vi "Multiplicate Number.vi"(8 "error in (no error)":errorcluster, 9 "Number 2":dbl, 10 "Number 1":dbl, 11 "Multiplication Actor in":refnum<class "Multiplication Actor.lvclass">) -> (0 "error out":errorcluster, 3 "Multiplication Actor out":refnum<class "Multiplication Actor.lvclass">)   [LabVIEW 2015, in "Multiplication Actor.lvclass"]
uses:
  Multiplication Actor.lvclass
  <vilib>/ActorFramework/Actor/Actor.lvclass/Actor.ctl
  Calculator Actor/Calculator Actor Messages/Update Multiplication Result Ref Msg/Update Multiplication Result Ref Msg.lvclass/Update Multiplication Result Ref Msg.ctl
  <vilib>/ActorFramework/Message Enqueuer/Message Enqueuer.lvclass/Message Enqueuer.ctl
  <vilib>/ActorFramework/Message Enqueuer/Enqueue.vi
  <vilib>/ActorFramework/Message Priority Queue/Priority Enqueue.vi
  Calculator Actor/Calculator Actor Messages/Update Multiplication Result Ref Msg/Update Multiplication Result Ref Msg.lvclass
  <vilib>/ActorFramework/Actor/Actor.lvclass
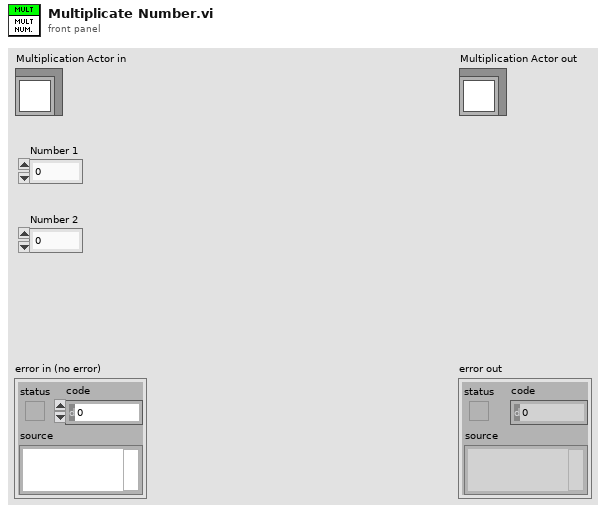
[diagram p1: front panel]
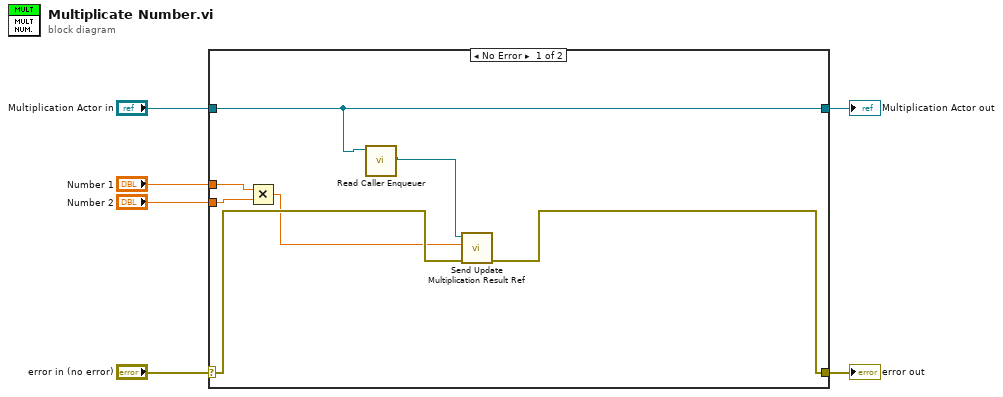
[diagram p0: block diagram]
diagram:
  n1 = case shown="No Error" "error in (no error)" {
    selector: "error in (no error)" -> [w13 w15]
    tunnel: [w12 w15] -> w5
    tunnel: [w8 w14] -> w3
    tunnel: "Multiplication Actor in" -> [w8 w14]
    tunnel: "Number 1" -> [w11 _]
    tunnel: "Number 2" -> [w10 _]
    frame No Error {
      n2 = Multiply(x=w11, y=w10) -> (x*y=w9:dbl)
      n3 = call <vilib>:"Read Caller Enqueuer.vi"("Actor"=w8) -> ("Caller Enqueuer"=w7:refnum<class "Message Enqueuer.lvclass">)  [unwired: 10 in]
      n4 = call "Send Update Multiplication Result Ref.vi"("error in (no error)"=w13, "Multiplication Result"=w9, "Message Enqueuer"=w7) -> ("error out"=w12:errorcluster)  [unwired: 7 in, 1 out]
    }
    frame Error {
    }
  }
  "error out" <- w5
  "Multiplication Actor out" <- w3
